vi "BRig_Host__Loop_Consumer_RunState__updatePlot__plotRange_get.vi"(5 "input_idx":i32[](array[numeric]), 7 "input_dataPlot":u16[][](array[numeric])) -> (2 "output_idxRange":i32[](array[numeric]))   [LabVIEW 2014]
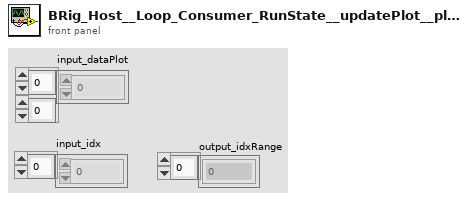
[diagram p1: front panel]
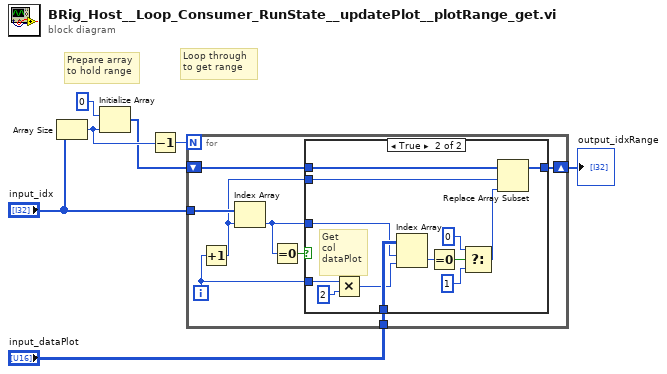
[diagram p0: block diagram]
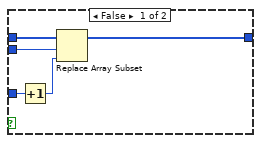
[diagram p2: hidden frame]
diagram:
  # "Loop through\nto get range"
  # "Prepare array\nto hold range"
  n1 = Array Size(array="input_idx") -> (size(s)=w6:i32)
  n2 = Initialize Array(0 ("element"), w6) -> (w4:i32[])
  n3 = Decrement(x=w6) -> (x-1=w5:i32)
  n4 = for {
    N: w5 -> [_]
    shift-right: [w12] -> w1
    shift-left: w4 -> [w13]
    tunnel: "input_idx" -> [w15]
    tunnel: "input_dataPlot" -> [w10]
    i -> [w8]
    n5 = Increment(x=w8) -> (x+1=w9:i32)
    n6 = Index Array(array=w15, index=w9) -> (element=w11:i32)
    n7 = Equal To 0?(x=w11) -> (x = 0?=w14:bool)
    n8 = case shown="True" w14 {
      tunnel: w13 -> [w20 w30]
      tunnel: [w19 w31] -> w12
      tunnel: w9 -> [w18 w29]
      tunnel: w11 -> [w17 w32]
      tunnel: w10 -> [_ w33]
      tunnel: w8 -> [_ w28]
      frame False {
        n9 = Increment(x=w17) -> (x+1=w16:i32)
        n10 = Replace Array Subset(array=w20, new element=w16, index=w18) -> (w19:i32[])
      }
      frame True {
        # "Get\ncol\ndataPlot"
        n11 = Multiply(x=w28, y=2) -> (x*y=w26:i32)
        n12 = Index Array(array=w33, index (row)=w32, index (col)=w26) -> (element=w24:u16)
        n13 = Equal To 0?(x=w24) -> (x = 0?=w25:bool)
        n14 = Select(t=0, s=w25, f=1) -> (s? t:f=w22:i32)
        n15 = Replace Array Subset(array=w30, new element=w22, index=w29) -> (w31:i32[])
      }
    }
  }
  "output_idxRange" <- w1
